vi "Method Info to Type.vi"(11 "Method Info":T1) -> (3 "Method Type":T2(ring))   [LabVIEW 2023]
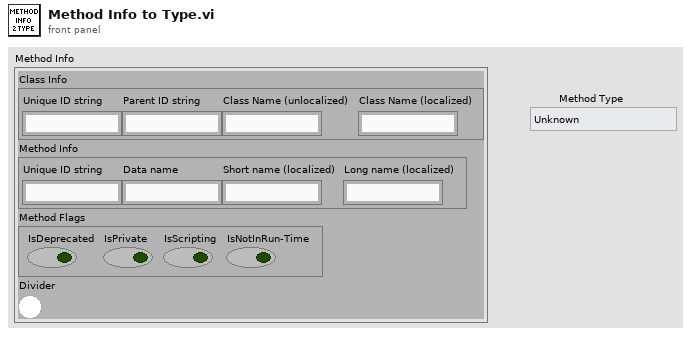
[diagram p1: front panel]
types:
  T1 = cluster{"Class Info":cluster{"Unique ID string":string, "Parent ID string":string, "Class Name (unlocalized)":string, "Class Name (localized)":string}, "Method Info":cluster{"Unique ID string":string, "Data name":string, "Short name (localized)":string, "Long name (localized)":string}, "Method Flags":cluster{"IsDeprecated":bool, "IsPrivate":bool, "IsScripting":bool, "IsNotInRun-Time":bool}, "Divider":bool}
  T2 = enum16{"Unknown", "Base", "Scripting", "Private", "Deprecated", "None", "Divider"}
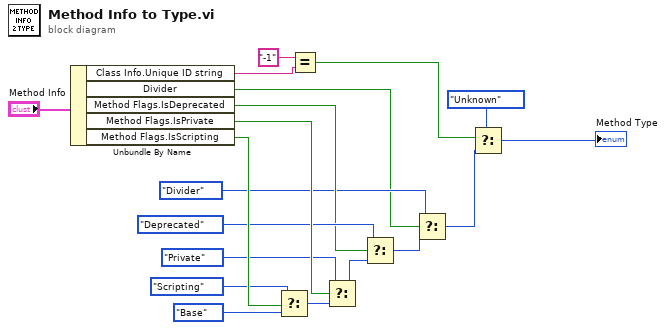
[diagram p0: block diagram]
diagram:
  n1 = Unbundle By Name("Method Info") -> ("Class Info.Unique ID string"=w9:string, "Divider"=w3:bool, "Method Flags.IsDeprecated"=w11:bool, "Method Flags.IsPrivate"=w18:bool, "Method Flags.IsScripting"=w19:bool)
  n2 = Select(t=T2."Scripting" ("Property Type"), s=w19, f=T2."Base" ("Property Type")) -> (s? t:f=w16:T2)
  n3 = Equal?(x="-1", y=w9) -> (x = y?=w7:bool)
  n4 = Select(t=T2."Private" ("Property Type"), s=w18, f=w16) -> (s? t:f=w10:T2)
  n5 = Select(t=T2."Deprecated" ("Property Type"), s=w11, f=w10) -> (s? t:f=w2:T2)
  n6 = Select(t=T2."Divider" ("Property Type"), s=w3, f=w2) -> (s? t:f=w1:T2)
  n7 = Select(t=T2."Unknown" ("Property Type"), s=w7, f=w1) -> (s? t:f=→"Method Type":T2)
